vi "Example- One Record at a Time.vi"() -> ()   [LabVIEW 2013]
doc: "This example shows the combined use of the Connection object and the Recordset object. We first create a connection object that retrieves all the rows from myTable. Then we use the recordset object to move through the records one at a time."
panel:
  out "EOF":bool
  in  "Next record":bool
  out "Record Data":string
  in  "SQL command":string
  in  "ConnectionString":string="DSN=myDB;"
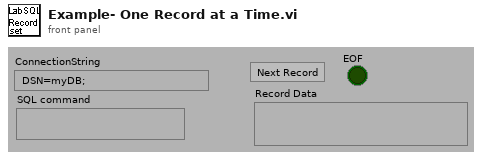
[diagram p1: front panel]
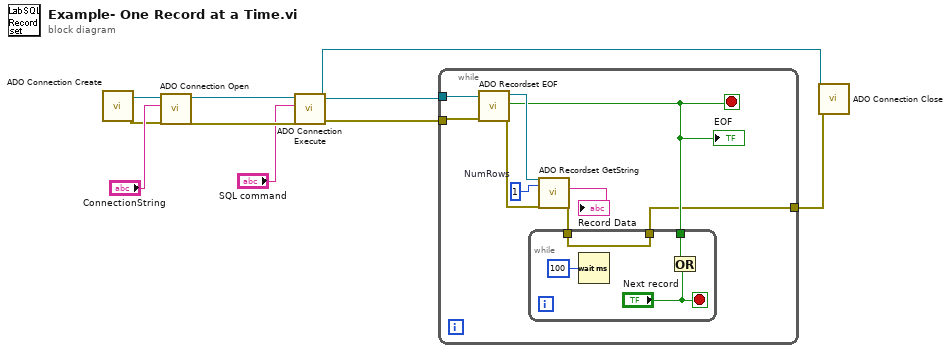
[diagram p0: block diagram]
diagram:
  n1 = call "ADO Connection Create.vi"() -> ("error out"=w9:errorcluster, "ADODB._Connection Out"=w8:refnum<k7>)  [unwired: 10 in]
  n2 = call "ADO Connection Open.vi"("error in (no error)"=w9, "ConnectionString"="ConnectionString", "ADODB._Connection In"=w8) -> ("error out"=w6:errorcluster, "ADODB._Connection Out"=w7:refnum<k7>)  [unwired: 7 in]
  n3 = call "ADO Connection Execute.vi"("error in (no error)"=w6, "CommandText"="SQL command", "ADODB._Connection In"=w7) -> ("error out"=w1:errorcluster, "RecordSet"=w2:refnum<k7>, "ADODB._Connection Out"=w3:refnum<k7>)  [unwired: 6 in]
  n4 = while {
    tunnel: [w11] -> w4
    tunnel: w1 -> [w18]
    tunnel: w2 -> [w19]
    stop <- w13 stop-if-true
    w12 = 1  # NumRows
    n5 = call "ADO Recordset EOF.vi"("error in (no error)"=w18, "ADODB._Recordset In"=w19) -> ("error out"=w16:errorcluster, "EOF"=w13:bool, "ADODB._Recordset Out"=w17:refnum<k7>)  [unwired: 7 in]
    "EOF" <- w13
    n6 = call "ADO Recordset GetString.vi"("ADODB._Recordset"=w17, "NumRows"=w12, "error in (no error)"=w16) -> ("GetString"=→"Record Data":string, "error out"=w14:errorcluster)  [unwired: 14 in, 1 out]
    n7 = while {
      tunnel: w13 -> [w20]
      tunnel: w14 -> [w22]
      tunnel: [w22] -> w11
      stop <- "Next record" stop-if-true
      n8 = Wait (ms)(milliseconds to wait=u32 100) -> ()  [unwired: 1 out]
      n9 = Or(x=w20, y="Next record") -> ()  [unwired: 1 out]
    }
  }
  n10 = call "ADO Connection Close.vi"("error in (no error)"=w4, "ADODB._Connection In"=w3) -> ()  [unwired: 8 in, 2 out]
